vi "CRYFind Max Step No in TS.vi"(8 "Inputflg":bool, 10 "Steps In":T1[](array[typedef]) {"Repeat State Array"."Start" format="%#_5g"; "Y dB ref" format="%.1f"; "Y data" items=["dB", "Lin"]; "Start" format="%#_5g"}, 11 "Required Count":i32) -> (3 "Num Array Out":i32[](array[numeric]))   [LabVIEW 2013]
uses:
  CRYSystem/Typedef Control/CRYStep.ctl
  CRYProject Editor Global.vi
panel:
  # "Get Max Number of Step No."
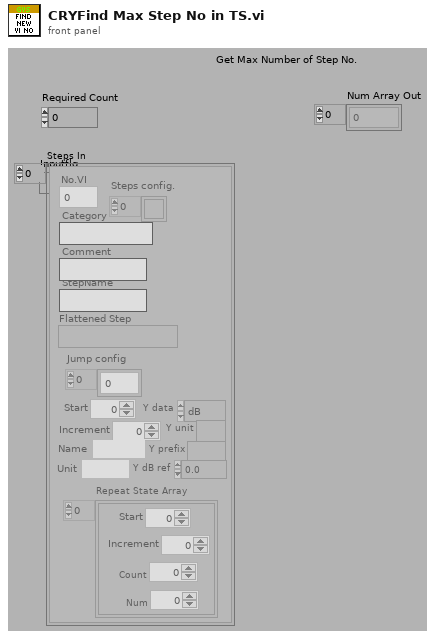
[diagram p1: front panel]
types:
  T1 = typedef "CRYStep.ctl" = cluster{"No.VI":i32, "Category":string, "StepName":string, "Seq setup flattened":string, "Comment":string, "Steps config.":bool[], "Jump config":i32[], "Start":dbl, "Increment":dbl, "Name":string, "Unit":string, "Y data":u16, "Y prefix":string, "Y dB ref":dbl, "Y unit":string, "Repeat State Array":cluster{"Start":dbl, "Increment":dbl, "Count":i32, "Num":i32}[]}
  T2 = typedef "CRYTS.ctl" = cluster{"No.TS":u16, "TS File Path":path, "TS Name":string, "EditStepName":string, "Steps":T1[], "New State":bool, "Change State":bool, "Flattened CurveLib Data":string, "Document Data":string, "EditStepNo":u16, "Operator Start File":string, "Sequence Type":string, "Sequence Language":string}
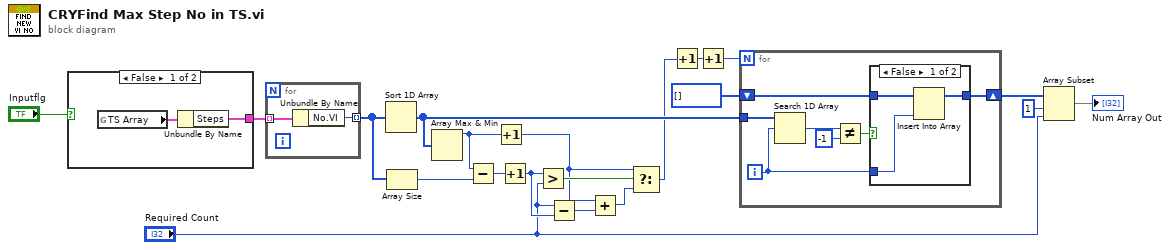
[diagram p0: block diagram]
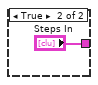
[diagram p2: hidden frame]
diagram:
  n1 = case shown="False" "Inputflg" {
    tunnel: [w22 "Steps In"] -> w5
    frame False {
      n2 = global read "CRYProject Editor Global.vi" "TS Array"() -> (w21:T2)
      n3 = Unbundle By Name(w21) -> ("Steps"=w22:T1[])
    }
    frame True {
    }
  }
  n4 = for {
    tunnel: w5 -> [w25] mode=indexing
    tunnel: [w24] -> w20 mode=indexing
    n5 = Unbundle By Name(w25) -> ("No.VI"=w24:i32)
  }
  n6 = Sort 1D Array(array=w20) -> (sorted array=w17:i32[])
  n7 = Array Size(array=w20) -> (size(s)=w12:i32)
  n8 = Array Max & Min(array=w17) -> (max value=w7:i32)  [unwired: 3 out]
  n9 = Subtract(x=w7, y=w12) -> (x-y=w16:i32)
  n10 = Increment(x=w7) -> (x+1=w6:i32)
  n11 = Increment(x=w16) -> (x+1=w14:i32)
  n12 = Greater?(x=w14, y="Required Count") -> (0:w15:bool)
  n13 = Subtract(x="Required Count", y=w14) -> (x-y=w11:i32)
  n14 = Add(x=w6, y=w11) -> (x+y=w13:i32)
  n15 = Select(t=w6, s=w15, f=w13) -> (s? t:f=w10:i32)
  n16 = Increment(x=w10) -> (x+1=w2:i32)
  n17 = Increment(x=w2) -> (x+1=w3:i32)
  n18 = for {
    N: w3 -> [_]
    tunnel: w17 -> [w29]
    shift-right: [w31] -> w18
    shift-left: i32[] [] ("Array") -> [w30]
    i -> [w26]
    n19 = Search 1D Array(1D array=w29, element=w26) -> (index of element=w28:i32)  [unwired: 1 in]
    n20 = Not Equal?(x=w28, y=-1) -> (x != y?=w32:bool)
    n21 = case shown="False" w32 {
      tunnel: w26 -> [w33 _]
      tunnel: [w34 w36] -> w31
      tunnel: w30 -> [w35 w36]
      frame False {
        n22 = Insert Into Array(array=w35, new element=w33) -> (w34:i32[])  [unwired: 1 in]
      }
      frame True {
      }
    }
  }
  n23 = Array Subset(array=w18, index=1, length="Required Count") -> (→"Num Array Out":i32[])
